vi "Interpolate 2D Scattered_Check Input 1D.vi"(0 "X In":dbl[](array[numeric]), 5 "Y In":dbl[](array[numeric]), 7 "Z In":dbl[](array[numeric]), 9 "Xi In":dbl[](array[numeric]), 11 "Yi In":dbl[](array[numeric])) -> (4 "X Out":dbl[](array[numeric]), 6 "Y Out":dbl[](array[numeric]), 8 "Z Out":dbl[](array[numeric]), 10 "Xi Out":dbl[](array[numeric]), 14 "error":i32, 15 "Yi Out":dbl[](array[numeric]))   [LabVIEW 2017, in "NI_AAL_Interpolation.lvlib"]
uses:
  <vilib>/gmath/NI_AAL_Interpolation.lvlib
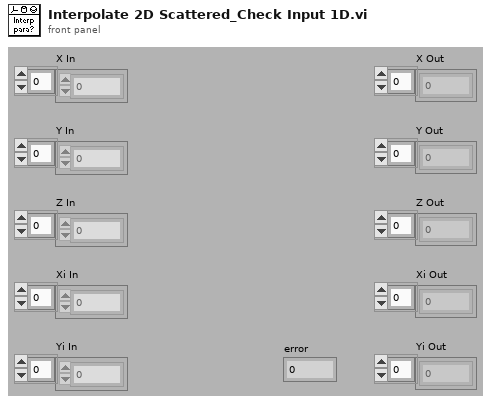
[diagram p1: front panel]
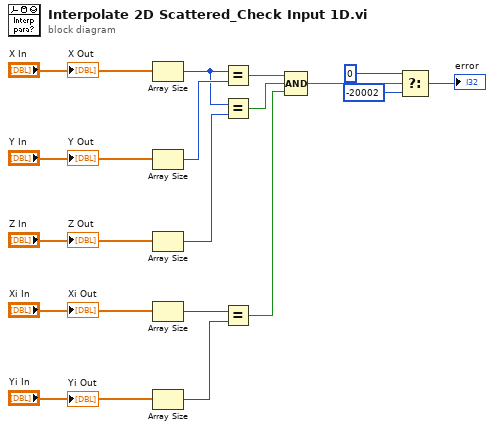
[diagram p0: block diagram]
diagram:
  n1 = Array Size(array="X In") -> (size(s)=w11:i32)
  n2 = Array Size(array="Y In") -> (size(s)=w12:i32)
  n3 = Array Size(array="Z In") -> (size(s)=w10:i32)
  n4 = Array Size(array="Xi In") -> (size(s)=w9:i32)
  n5 = Array Size(array="Yi In") -> (size(s)=w8:i32)
  n6 = Equal?(x=w11, y=w12) -> (x = y?=w7:bool)
  n7 = Equal?(x=w11, y=w10) -> (x = y?=w6:bool)
  n8 = Equal?(x=w9, y=w8) -> (x = y?=w5:bool)
  n9 = Compound Arithmetic op=AND(w7, w6, w5) -> (w4:bool)
  n10 = Select(t=0, s=w4, f=-20002) -> (s? t:f=→"error":i32)
  "X Out" <- "X In"
  "Y Out" <- "Y In"
  "Z Out" <- "Z In"
  "Xi Out" <- "Xi In"
  "Yi Out" <- "Yi In"
